vi "CLUSTERComplex.vi"() -> ()   [LabVIEW 2014]
doc: "This function takes a cluster that contains a DBL, string, and array of I32 (in that order) as input (the string and array items are pointers to data outside of the structure). It squares the value of the DBL, reverses the input string and concatenates the reversed string to the original string, and doubles the value of each element in the array. The result is returned in output.\n\nFor information on the data types used for the DLL function, right-click on the Call Library Function node and choose Configure."
uses:
  CLF_Example.dll
panel:
  out "output":T1
  in  "input":T1={"DBL"=10.0, "String (No Character Limit)"="abcd", "Array (No Element Limit)"=[10, 100]}
  # "See the block diagram for more information."
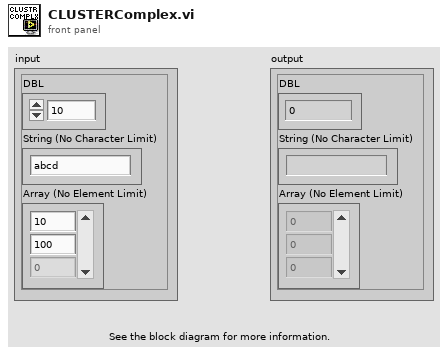
[diagram p1: front panel]
types:
  T1 = cluster{"DBL":dbl, "String (No Character Limit)":string, "Array (No Element Limit)":i32[]}
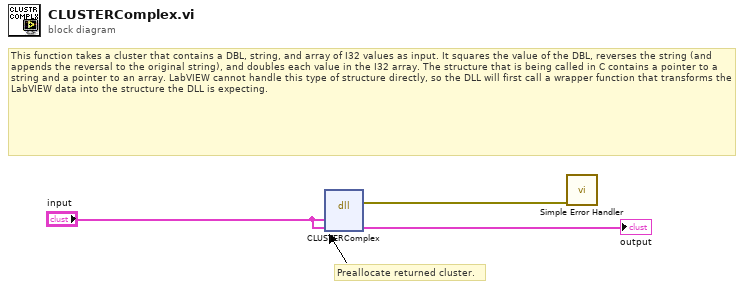
[diagram p0: block diagram]
diagram:
  # "Preallocate returned cluster."
  # "This function takes a cluster that contains a DBL, string, and array of I32 values as input. It squares the value of the DBL, reverses the string (and appends the reversal to the original string), and doubles each value in the I32 array. The structure that is being called in C contains a pointer to a string and a pointer to an array. LabVIEW cannot handle this type of structure directly, so the DLL will first call a wrapper function that transforms the LabVIEW data into the structure the DLL is expecting."
  n1 = dll-call lib="e:/builds/penguin/labview/branches/2014/dev/dist/examples/Connectivity/Libraries and Executables/DLL Calling VIs/CLF_Example**.*" fn="CLUSTERComplex"("input"="input", "output"="input") -> (error out=w1:errorcluster, "output"=→"output":T1)  [unwired: 4 in, 2 out]
  n2 = call <vilib>:"Simple Error Handler.vi"("error in (no error)"=w1) -> ()  [unwired: 4 in, 5 out]
